vi "LookForPostInstHold.vi"(6 "Initialize?":bool, 7 "Touch lines":T2={"Home touch"=0, "Touch 1"=1, "Touch 2"=2, "Touch 3"=3, "Touch 4"=4}, 9 "Post-I \nbounce-off":cluster{"Fix":dbl, "Rnd":dbl}={"Fix"=0.3, "Rnd"=0.0} caption="Allowed\nbounce-off" {"Rnd" format="%.4f"; "Fix" format="%_4g"}, 10 "Post-I hold":cluster{"Fix":dbl, "Rnd":dbl}={"Fix"=0.5, "Rnd"=0.5} {"Rnd" format="%.4f"; "Fix" format="%.4f"}, 11 "DI Task":refnum<k21>) -> (0 "Last trial successful?":bool, 3 "Go to stage":T1(ring))   [LabVIEW 2010]
panel:
  # "+"
  # "+"
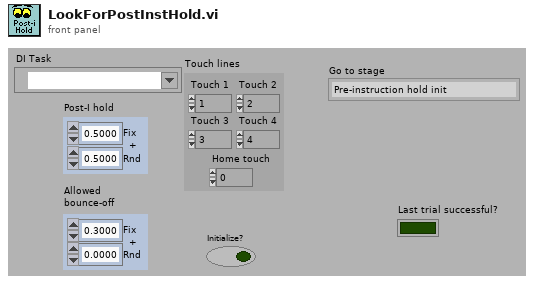
[diagram p1: front panel]
types:
  T1 = enum16{"Pre-instruction hold init", "Pre-instruction hold", "Instruction init", "Instruction", "Post-instruction hold init", "Post-instruction hold", "Target capture init", "Target capture", "Target hold init", "Target hold", "Reward stage", "Intertrial"}
  T2 = cluster{"Home touch":i16, "Touch 1":i16, "Touch 2":i16, "Touch 3":i16, "Touch 4":i16}
  T3 = enum16{"Home", "Touch 1", "Touch 2", "Touch 3", "Touch 4", "None"}
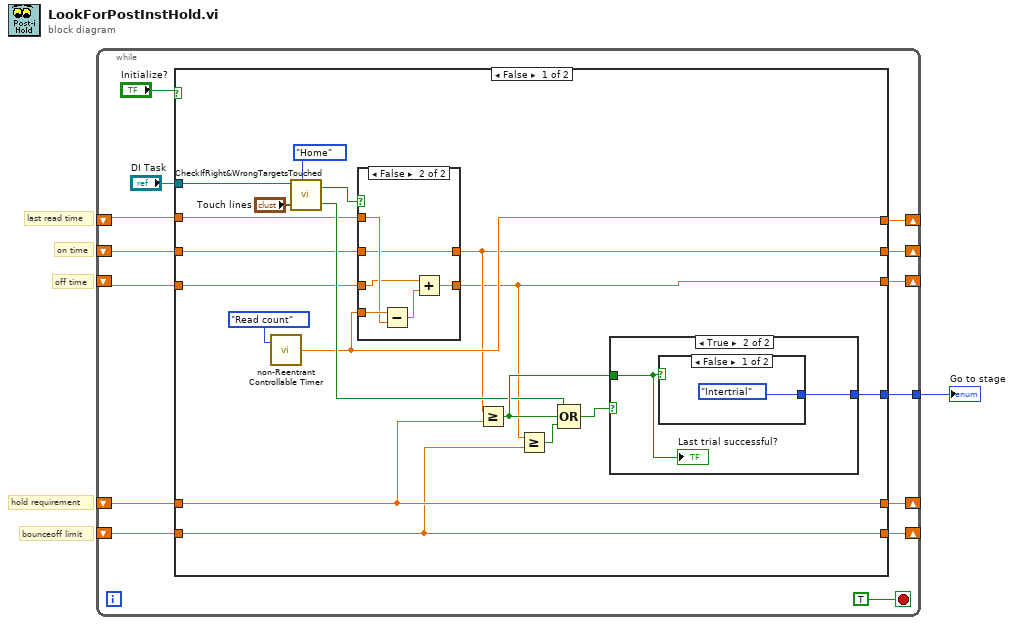
[diagram p0: block diagram]
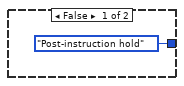
[diagram p2: hidden frame]
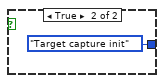
[diagram p3: hidden frame]
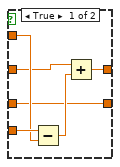
[diagram p4: hidden frame]
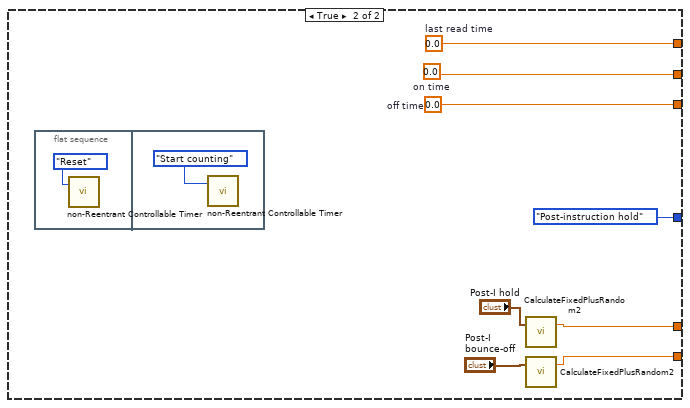
[diagram p5: hidden frame]
diagram:
  # "bounceoff limit"
  # "hold requirement"
  # "off time"
  # "on time"
  # "last read time"
  n1 = while {
    tunnel: [w14] -> w1
    shift-right: [w12] -> _
    shift-left: _ -> [w9]
    shift-right: [w11] -> _
    shift-left: _ -> [w8]
    shift-right: [w10] -> _
    shift-left: _ -> [w7]
    shift-right: [w6] -> _
    shift-left: _ -> [w4]
    shift-right: [w5] -> _
    shift-left: _ -> [w3]
    stop <- TRUE stop-if-true
    n2 = case shown="False" "Initialize?" {
      tunnel: [w33 T1."Post-instruction hold" ("Current stage")] -> w14
      tunnel: [w22 w58] -> w12
      tunnel: [w21 w57] -> w11
      tunnel: [w20 w56] -> w10
      tunnel: w9 -> [w25 _]
      tunnel: w8 -> [w24 _]
      tunnel: w7 -> [w23 _]
      tunnel: [w18 w52] -> w6
      tunnel: [w17 w51] -> w5
      tunnel: w4 -> [w18 _]
      tunnel: w3 -> [w17 _]
      tunnel: "DI Task" -> [w16 _]
      frame False {
        n3 = call "non-Reentrant Controllable Timer.vi"("Enum"=enum16{"Start counting", "Read count", "Reset"}."Read count") -> ("Time out"=w22:dbl)  [unwired: 1 in]
        n4 = call "CheckIfRight&WrongTargetsTouched.vi"("Target"=T3."Home", "Touch sensor lines"="Touch lines", "DI Task"=w16) -> ("Wrong target touched?"=w28:bool, "Target touched?"=w30:bool)  [unwired: 3 in]
        n5 = case shown="False" w30 {
          tunnel: w24 -> [w39 w48]
          tunnel: w23 -> [w41 w45]
          tunnel: w22 -> [w43 w50]
          tunnel: w25 -> [w42 w49]
          tunnel: [w41 w47] -> w20
          tunnel: [w40 w48] -> w21
          frame True {
            n6 = Subtract(x=w43, y=w42) -> (x-y=w44:dbl)
            n7 = Add(x=w39, y=w44) -> (x+y=w40:dbl)
          }
          frame False {
            n8 = Subtract(x=w50, y=w49) -> (x-y=w46:dbl)
            n9 = Add(x=w45, y=w46) -> (x+y=w47:dbl)
          }
        }
        n10 = Greater Or Equal?(x=w21, y=w18) -> (x >= y?=w32:bool)
        n11 = Greater Or Equal?(x=w20, y=w17) -> (x >= y?=w29:bool)
        n12 = Compound Arithmetic op=OR(w28, w32, w29) -> (w19:bool)
        n13 = case shown="True" w19 {
          tunnel: [T1."Post-instruction hold" ("Current stage") w36] -> w33
          tunnel: w32 -> [_ w35]
          frame False {
          }
          frame True {
            n14 = case shown="False" w35 {
              tunnel: [T1."Intertrial" ("Current stage") T1."Target capture init" ("Current stage")] -> w36
              frame False {
              }
              frame True {
              }
            }
            "Last trial successful?" <- w35
          }
        }
      }
      frame True {
        w58 = 0.0  # last read time
        w56 = 0.0  # off time
        w57 = 0.0  # on time
        n15 = flat-sequence {
          frame #0 {
            n16 = call "non-Reentrant Controllable Timer.vi"("Enum"=enum16{"Start counting", "Read count", "Reset"}."Reset") -> ()  [unwired: 1 in, 1 out]
          }
          frame #1 {
            n17 = call "non-Reentrant Controllable Timer.vi"("Enum"=enum16{"Start counting", "Read count", "Reset"}."Start counting") -> ()  [unwired: 1 in, 1 out]
          }
        }
        n18 = call "CalculateFixedPlusRandom2.vi"("Component times"="Post-I hold") -> ("Composite time"=w52:dbl)  [unwired: 1 in, 1 out]
        n19 = call "CalculateFixedPlusRandom2.vi"("Component times"="Post-I \nbounce-off") -> ("Composite time"=w51:dbl)  [unwired: 1 in, 1 out]
      }
    }
  }
  "Go to stage" <- w1
